vi "GCalculator.vi"() -> ()   [LabVIEW 2015]
panel:
  out "Hacim":dbl
  out "Alan":dbl
  out "Cevre":dbl
  in  "h":dbl
  in  "y":dbl
  in  "x":dbl
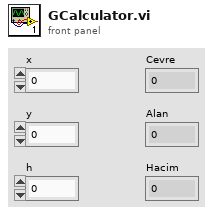
[diagram p1: front panel]
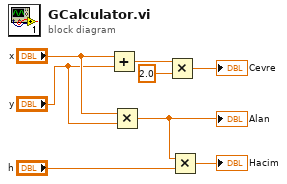
[diagram p0: block diagram]
diagram:
  n1 = Add(x="x", y="y") -> (x+y=w8:dbl)
  n2 = Multiply(x="x", y="y") -> (x*y=w2:dbl)
  "Alan" <- w2
  n3 = Multiply(x=w8, y=2.0) -> (x*y=→"Cevre":dbl)
  n4 = Multiply(x=w2, y="h") -> (x*y=→"Hacim":dbl)
